vi "error too far sub.vi"(1 "current position":dbl) -> (0 "String":string)   [LabVIEW 2018]
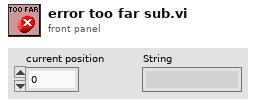
[diagram p1: front panel]
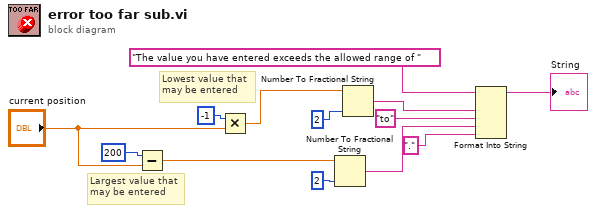
[diagram p0: block diagram]
diagram:
  # "Largest value that\nmay be entered"
  # "Lowest value that\nmay be entered"
  n1 = Subtract(x=200, y="current position") -> (x-y=w7:dbl)
  n2 = Multiply(x=-1, y="current position") -> (x*y=w10:dbl)
  n3 = Number To Fractional String(number=w7, precision (6)=2) -> (F-format string=w8:string)  [unwired: 2 in]
  n4 = Number To Fractional String(number=w10, precision (6)=2) -> (F-format string=w9:string)  [unwired: 2 in]
  n5 = Format Into String(initial string="The value you have entered exceeds the allowed range of ", w9, "to", w8, ".") -> (resulting string=→"String":string)  [unwired: 2 in, 1 out]
